vi "McsaIntializeDFScript.vi"(8 "error in (no error)":errorcluster) -> (0 "error out":errorcluster)   [LabVIEW 2017]
uses:
  <vilib>/addons/InsightCM/Devices/Shared/Common/DataFlow/controls/Type.ctl
  <vilib>/addons/InsightCM/Devices/Shared/Common/Trigger/Trigger.lvlib
  <vilib>/addons/InsightCM/Devices/Shared/Common/DataAccumulator/DataAccumulator.lvlib
  <vilib>/addons/InsightCM/Devices/Shared/Common/DataFlow/DataFlow.lvlib
  <vilib>/addons/InsightCM/Devices/Shared/Common/FileFlow/FileFlow.lvlib
  <vilib>/addons/InsightCM/Devices/Shared/Common/OpState/OpState.lvlib
  <vilib>/addons/InsightCM/Devices/Shared/Common/TrendAlarm/TrendAlarm.lvlib
  <vilib>/addons/InsightCM/Devices/Shared/Mcsa/McsaVirtualChannel/McsaVirtualChannel.lvlib
  <vilib>/addons/InsightCM/Devices/Shared/Mcsa/McsaAnalysisHighRate/McsaAnalysisHighRate.lvlib
  <vilib>/addons/InsightCM/Devices/Shared/Mcsa/McsaAnalysisLowRate/McsaAnalysisLowRate.lvlib
  <vilib>/addons/InsightCM/Devices/Shared/Mcsa/McsaAnalysisLowUpdate/McsaAnalysisLowUpdate.lvlib
  <vilib>/addons/InsightCM/Devices/Shared/Mcsa/McsaStartupAnalysis/McsaStartupAnalysis.lvlib
  <vilib>/addons/InsightCM/Devices/Shared/Mcsa/McsaDataEventCreator/McsaDataEventCreator.lvlib
  <vilib>/addons/InsightCM/Devices/Shared/Mcsa/McsaTestPanel/McsaTestPanel.lvlib
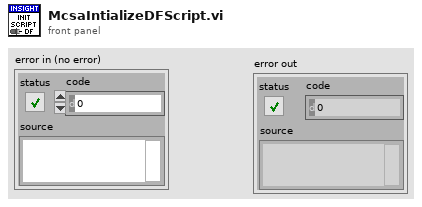
[diagram p1: front panel]
types:
  T1 = typedef "DataFlow.lvlib/Type.ctl" = enum16{"High Rate", "Low Rate", "Burst Mode"}
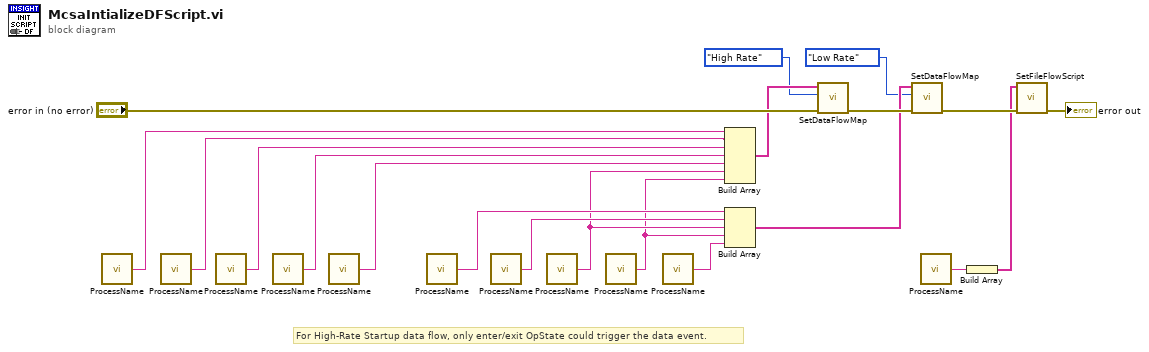
[diagram p0: block diagram]
diagram:
  # "For High-Rate Startup data flow, only enter/exit OpState could trigger the data event."
  n1 = call <vilib>:"ProcessName.vi"() -> ("ProcessName"=w14:string)  [unwired: 5 in]
  n2 = call <vilib>:"ProcessName.vi"() -> ("ProcessName"=w12:string)  [unwired: 5 in]
  n3 = call <vilib>:"ProcessName.vi"() -> ("ProcessName"=w3:string)  [unwired: 5 in]
  n4 = call <vilib>:"ProcessName.vi"() -> ("process name"=w15:string)  [unwired: 5 in]
  n5 = call <vilib>:"ProcessName.vi"() -> ("process name"=w16:string)  [unwired: 5 in]
  n6 = call <vilib>:"ProcessName.vi"() -> ("ProcessName"=w10:string)  [unwired: 5 in]
  n7 = call <vilib>:"ProcessName.vi"() -> ("process name"=w8:string)  [unwired: 5 in]
  n8 = call <vilib>:"ProcessName.vi"() -> ("process name"=w7:string)  [unwired: 5 in]
  n9 = call <vilib>:"ProcessName.vi"() -> ("process name"=w6:string)  [unwired: 5 in]
  n10 = call <vilib>:"ProcessName.vi"() -> ("process name"=w5:string)  [unwired: 5 in]
  n11 = Build Array(w14, w12, w3, w15, w16, w7, w6) -> (w11:string[])
  n12 = Build Array(w10, w8, w7, w6, w5) -> (w13:string[])
  n13 = call <vilib>:"SetDataFlowMap.vi"("error in (no error)"="error in (no error)", "type"=Type."High Rate", "Dataflow script"=w11) -> ("error out"=w18:errorcluster)  [unwired: 8 in]
  n14 = call <vilib>:"SetDataFlowMap.vi"("error in (no error)"=w18, "type"=Type."Low Rate", "Dataflow script"=w13) -> ("error out"=w17:errorcluster)  [unwired: 8 in]
  n15 = call <vilib>:"ProcessName.vi"() -> ("ProcessName"=w9:string)  [unwired: 5 in]
  n16 = Build Array(w9) -> (w4:string[])
  n17 = call <vilib>:"SetFileFlowScript.vi"("error in (no error)"=w17, "Fileflow script"=w4) -> ("error out"=→"error out":errorcluster)  [unwired: 9 in]
